vi "MainUI.vi"(8 "error in (no error)":errorcluster) -> (0 "error out":errorcluster)   [LabVIEW 2017]
doc: "Use this template to build a VI to use as a subVI."
panel:
  out "String 16":string
  out "String 15":string
  out "String 14":string
  out "String 13":string
  out "String 12":string
  out "String 11":string
  out "String 10":string
  out "String 9":string
  out "String 8":string
  out "String 7":string
  out "String 6":string
  out "String 5":string
  out "String 4":string
  out "String 3":string
  out "String 2":string
  out "String":string
  out "LogTextBox":string
  out "CurrentActionText":string
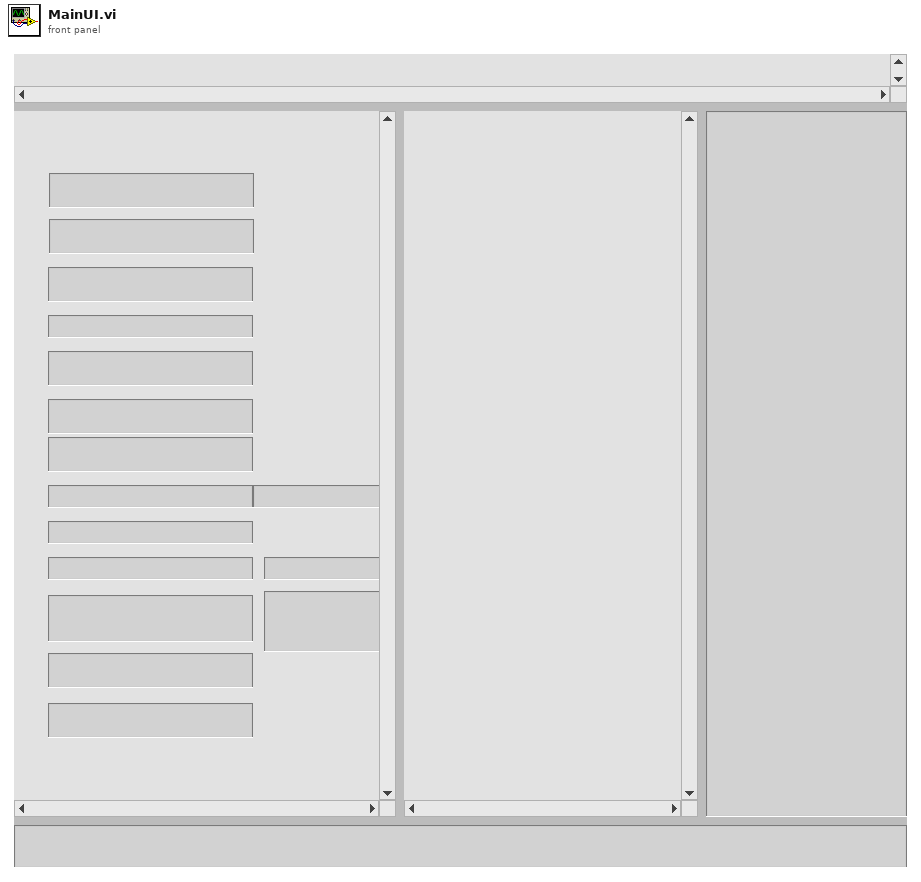
[diagram p1: front panel]
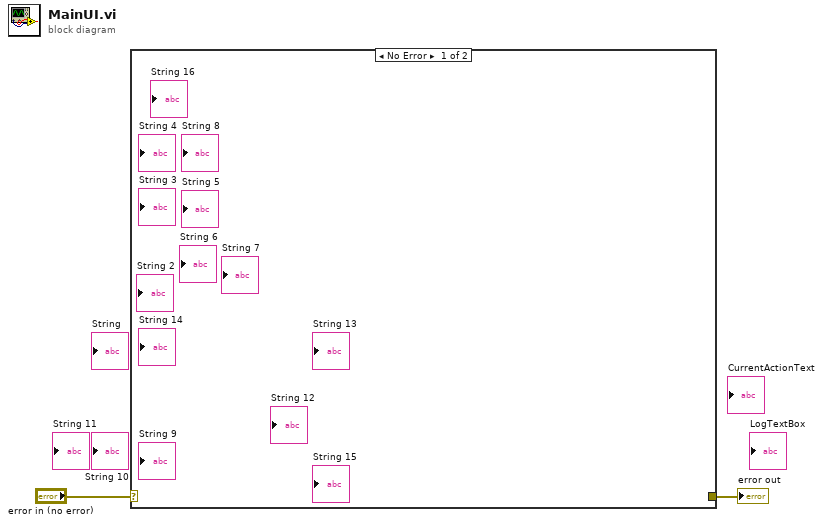
[diagram p0: block diagram]
diagram:
  n1 = case shown="No Error" "error in (no error)" {
    selector: "error in (no error)" -> [_ w3]
    tunnel: [_ w3] -> w1
    frame No Error {
    }
    frame Error {
    }
  }
  "error out" <- w1
